vi "median3.vi"(6 "Reset":bool, 10 "In":sgl[](array[numeric]) format="%#_3p") -> (2 "Out":sgl[](array[numeric]) format="%#_3p")   [LabVIEW 2013]
panel:
  # "Order 3 median filter on vector signal.  The median is computed independently for each signal dimension."
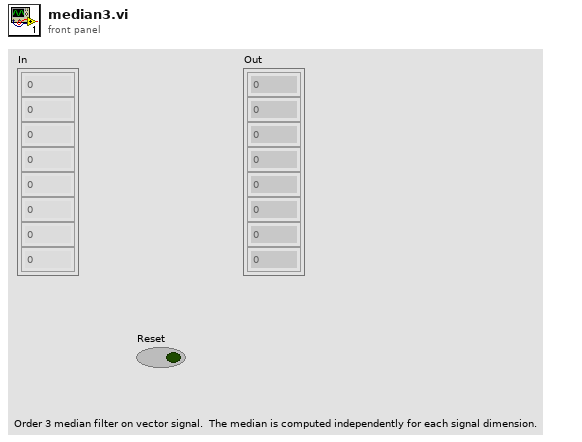
[diagram p1: front panel]
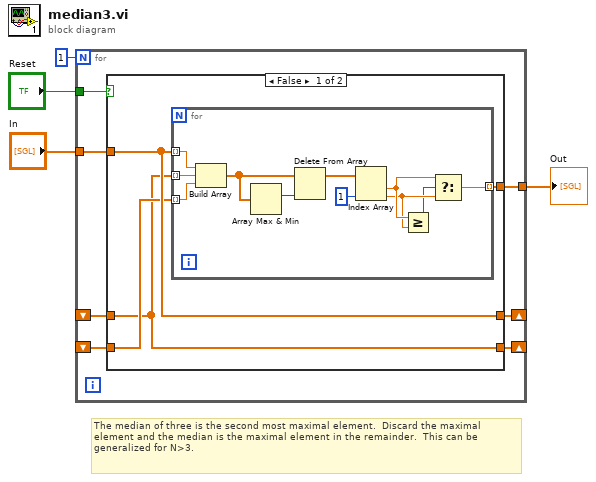
[diagram p0: block diagram]
diagram:
  # "The median of three is the second most maximal element.  Discard the maximal element and the median is the maximal element in the remainder.  This can be generalized for N>3."
  n1 = for {
    N: 1 -> [_]
    shift-right: [w10] -> _
    shift-left: _ -> [w7]
    shift-right: [w8] -> _
    shift-left: _ -> [w6]
    tunnel: "In" -> [w9]
    tunnel: "Reset" -> [w11]
    tunnel: [w5] -> w1
    n2 = case shown="False" w11 {
      tunnel: [w15 w27] -> w10
      tunnel: w9 -> [w15 w27]
      tunnel: [w13 w27] -> w8
      tunnel: w7 -> [w13 _]
      tunnel: w6 -> [w14 _]
      tunnel: [w12 w27] -> w5
      frame False {
        n3 = for {
          tunnel: w15 -> [w26] mode=indexing
          tunnel: w13 -> [w25] mode=indexing
          tunnel: w14 -> [w24] mode=indexing
          tunnel: [w16] -> w12 mode=indexing
          n4 = Build Array(w26, w25, w24) -> (w23:sgl[])
          n5 = Array Max & Min(array=w23) -> (max index (indices)=w22:i32)  [unwired: 3 out]
          n6 = Delete From Array(array=w23, index=w22) -> (array with subset deleted=w21:sgl[])  [unwired: 1 in, 1 out]
          n7 = Index Array(array=w21, index #2=1 ("index")) -> (element #1=w19:sgl, element #2=w18:sgl)  [unwired: 1 in]
          n8 = Greater Or Equal?(x=w19, y=w18) -> (x >= y?=w17:bool)
          n9 = Select(t=w19, s=w17, f=w18) -> (s? t:f=w16:sgl)
        }
      }
      frame True {
        # "Reset"
      }
    }
  }
  "Out" <- w1
